vi "Login Rmb User.vi"(8 "error in (no error)":errorcluster, 10 "rmb user":bool, 11 "[C] User Management in":refnum<class "[C] User Management.lvclass">) -> (0 "error out":errorcluster, 3 "[C] User Management out":refnum<class "[C] User Management.lvclass">)   [LabVIEW 2020, in "[C] User Management.lvlib" / "[C] User Management.lvclass"]
uses:
  [C] User Management.lvclass
  [C] User Management.lvclass/[C] User Management.ctl
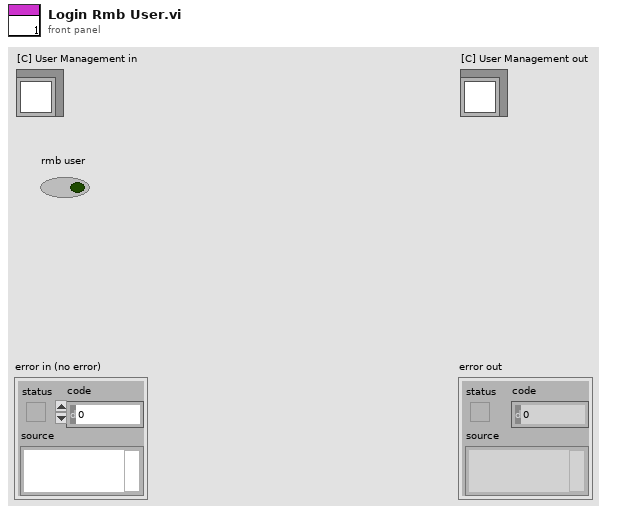
[diagram p1: front panel]
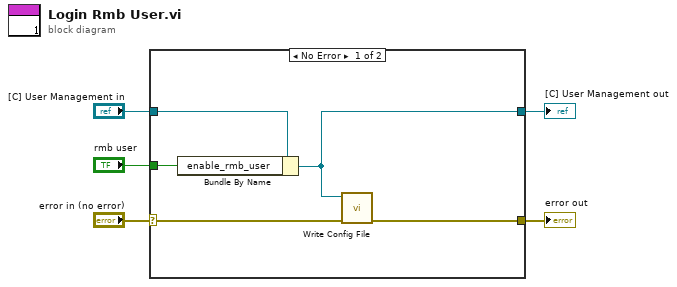
[diagram p0: block diagram]
diagram:
  n1 = case shown="No Error" "error in (no error)" {
    selector: "error in (no error)" -> [w8 w12]
    tunnel: [w6 w12] -> w2
    tunnel: "[C] User Management in" -> [w10 w11]
    tunnel: [w7 w11] -> w4
    tunnel: "rmb user" -> [w9 _]
    frame No Error {
      n2 = Bundle By Name(cluster=w10, "enable_rmb_user"=w9) -> (w7:refnum<class "[C] User Management.lvclass">)
      n3 = call "Write Config File.vi"("error in (no error)"=w8, "[C] User Management in"=w7) -> ("error out"=w6:errorcluster)  [unwired: 8 in, 1 out]
    }
    frame Error {
    }
  }
  "error out" <- w2
  "[C] User Management out" <- w4
